vi "getCurrentCmd.vi"(8 "error in (no error)":errorcluster, 11 "Subsystem in":refnum<class "Subsystem.lvclass">) -> (0 "error out":errorcluster, 2 "Command.lvclass":refnum<class "Command.lvclass">, 3 "Subsystem out":refnum<class "Subsystem.lvclass">)   [LabVIEW 2017, in "Subsystem.lvclass"]
uses:
  <userlib>/836-Library/Robot/Subsystem/Subsystem.lvclass
  <userlib>/836-Library/Robot/Command/Command.lvclass
  <userlib>/836-Library/Robot/Subsystem/Subsystem.lvclass/Subsystem.ctl
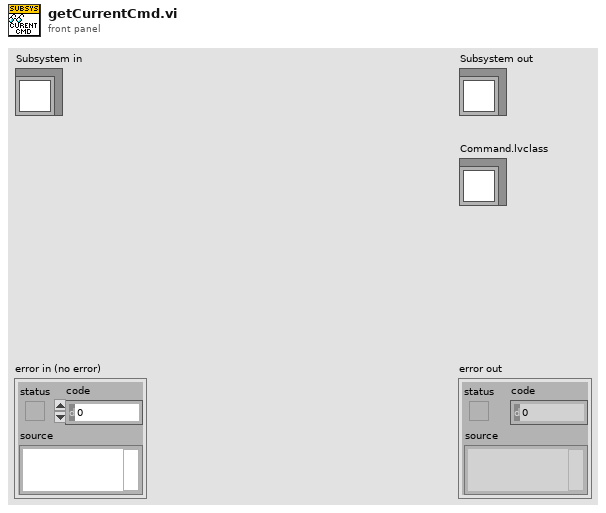
[diagram p1: front panel]
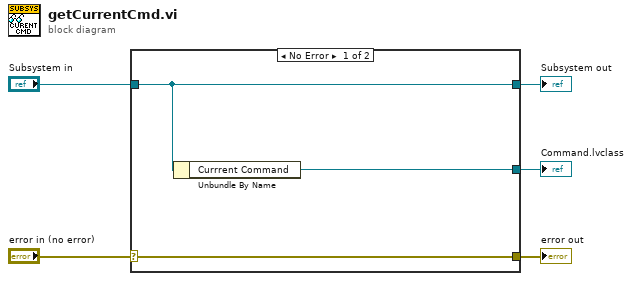
[diagram p0: block diagram]
diagram:
  n1 = case shown="No Error" "error in (no error)" {
    selector: "error in (no error)" -> [w8 w9]
    tunnel: [w8 w9] -> w4
    tunnel: [w7 w10] -> w2
    tunnel: "Subsystem in" -> [w7 w10]
    tunnel: [w6 _] -> w1
    frame No Error {
      n2 = Unbundle By Name(w7) -> ("Currrent Command"=w6:refnum<class "Command.lvclass">)
    }
    frame Error {
    }
  }
  "error out" <- w4
  "Subsystem out" <- w2
  "Command.lvclass" <- w1
